vi "Reef Tele Align.vi"(1 "Robot Velocities":T2={"X Velocity"=-0.05891453742478221, "Y Velocity"=0.05531455287310416, "Rotational \nVelocity"=-0.0}, 2 "PigeonIMUDevRef":T3={"DeviceStatus"={"status"=FALSE, "code"=0, "source"=""}, "Device Number"=21, "Type"=352321536, "Device ID"=352321557, "Handle"=27000480, "UsageFrame"=0, "Library Path"=path "libCTRE_PhoenixCCI.so"} {"Type" items=["CAN"=352321536, "TalonSRX"=33554432]}) -> (0 "Robot Velocities":T2={"X Velocity"=-0.05891453742478221, "Y Velocity"=0.05531455287310416, "Rotational \nVelocity"=-0.0})   [LabVIEW 2023]
uses:
  <vilib>/Rock Robotics/WPI/ThirdParty/Phoenix-LabVIEW/Pigeon IMU/CTRE_PigeonIMU_DeviceRef.ctl
  <vilib>/Rock Robotics/WPI/ThirdParty/Phoenix-LabVIEW/Pigeon IMU/CTRE_PigeonIMU_ConnectionType.ctl
  swerve/Type Definitions/Data/Robot Velocities.ctl
  <vilib>/Rock Robotics/Network Tables/NT Read Numeric Array.vi
  <vilib>/Rock Robotics/WPI/ThirdParty/Phoenix-LabVIEW/Pigeon IMU/CTRE_PigeonIMU_GetYPR.vi
panel:
  in  "F Value X":dbl=0.8 format="%.2f"
  in  "FeedFwd Value":dbl=0.8 format="%.2f"
  out "Limelight Value":dbl[](array[numeric])=[0.09069335352360994, 0.2555777244634621, -1.0504762124767997, -1.0032725806064795, -8.759387018378728, -0.17873698055030388]
  in  "Setpoint Y":dbl=1.0
  in  "Setpoint X":dbl
  in  "Deadband Y":dbl=0.1
  in  "PID Y":T1={"proportional gain (Kp)"=0.2, "integral time (Ki)"=0.0, "derivative time (Kd)"=0.0} {"derivative time (Kd)" format="%.3f"; "integral time (Ki)" format="%.3f"; "proportional gain (Kp)" format="%.3f"}
  out "Err/Out Chart 2":cluster{dbl, dbl}(graph)={2.1086785037111793, 0.6326035511133538}
  out "SP/PV Chart 2":cluster{"setpoint":dbl, "process variable":dbl}(graph)={"setpoint"=1.0, "process variable"=-1.1086785037111793}
  out "SP/PV Chart":cluster{"setpoint":dbl, "process variable":dbl}(graph)={"setpoint"=0.0, "process variable"=0.10840384468168587}
  out "Err/Out Chart":cluster{dbl, dbl}(graph)={-0.10840384468168587, -0.03252115340450576}
  in  "PID X":T1={"proportional gain (Kp)"=0.2, "integral time (Ki)"=0.0, "derivative time (Kd)"=0.0} {"derivative time (Kd)" format="%.3f"; "integral time (Ki)" format="%.3f"; "proportional gain (Kp)" format="%.3f"}
  in  "Deadband X":dbl=0.075
  out "Yaw Pitch Roll":cluster{"Yaw":dbl, "Pitch":dbl, "Roll":dbl}
  out "X":dbl=0.09069335352360994
  out "Y":dbl=-1.0504762124767997
  # "Y Errors"
  # "X Errors"
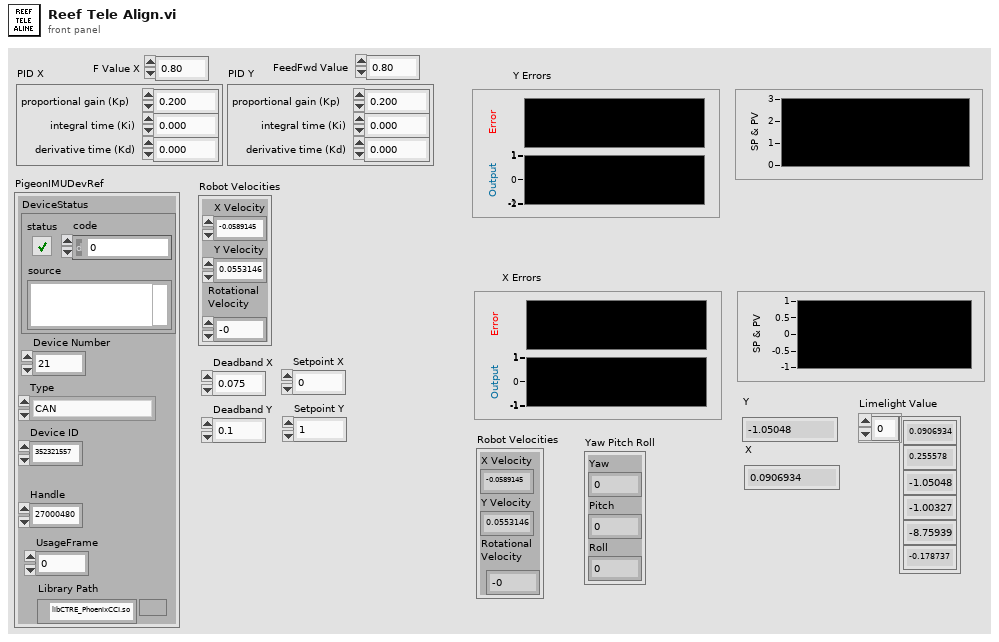
[diagram p1: front panel]
types:
  T1 = cluster{"proportional gain (Kp)":dbl, "integral time (Ki)":dbl, "derivative time (Kd)":dbl}
  T2 = typedef "Robot Velocities.ctl" = cluster{"X Velocity":dbl, "Y Velocity":dbl, "Rotational \nVelocity":dbl}
  T3 = typedef "CTRE_PigeonIMU_DeviceRef.ctl" = cluster{"DeviceStatus":errorcluster, "Device Number":u8, "Type":T4, "Device ID":u32, "Handle":u64, "UsageFrame":u32, "Library Path":path}
  T4 = typedef "CTRE_PigeonIMU_ConnectionType.ctl" = u32
  T5 = cluster{"value[0]":dbl, "value[1]":dbl, "value[2]":dbl, "value[3]":dbl, "value[4]":dbl, "value[5]":dbl, "value[6]":dbl, "value[7]":dbl, "value[8]":dbl}
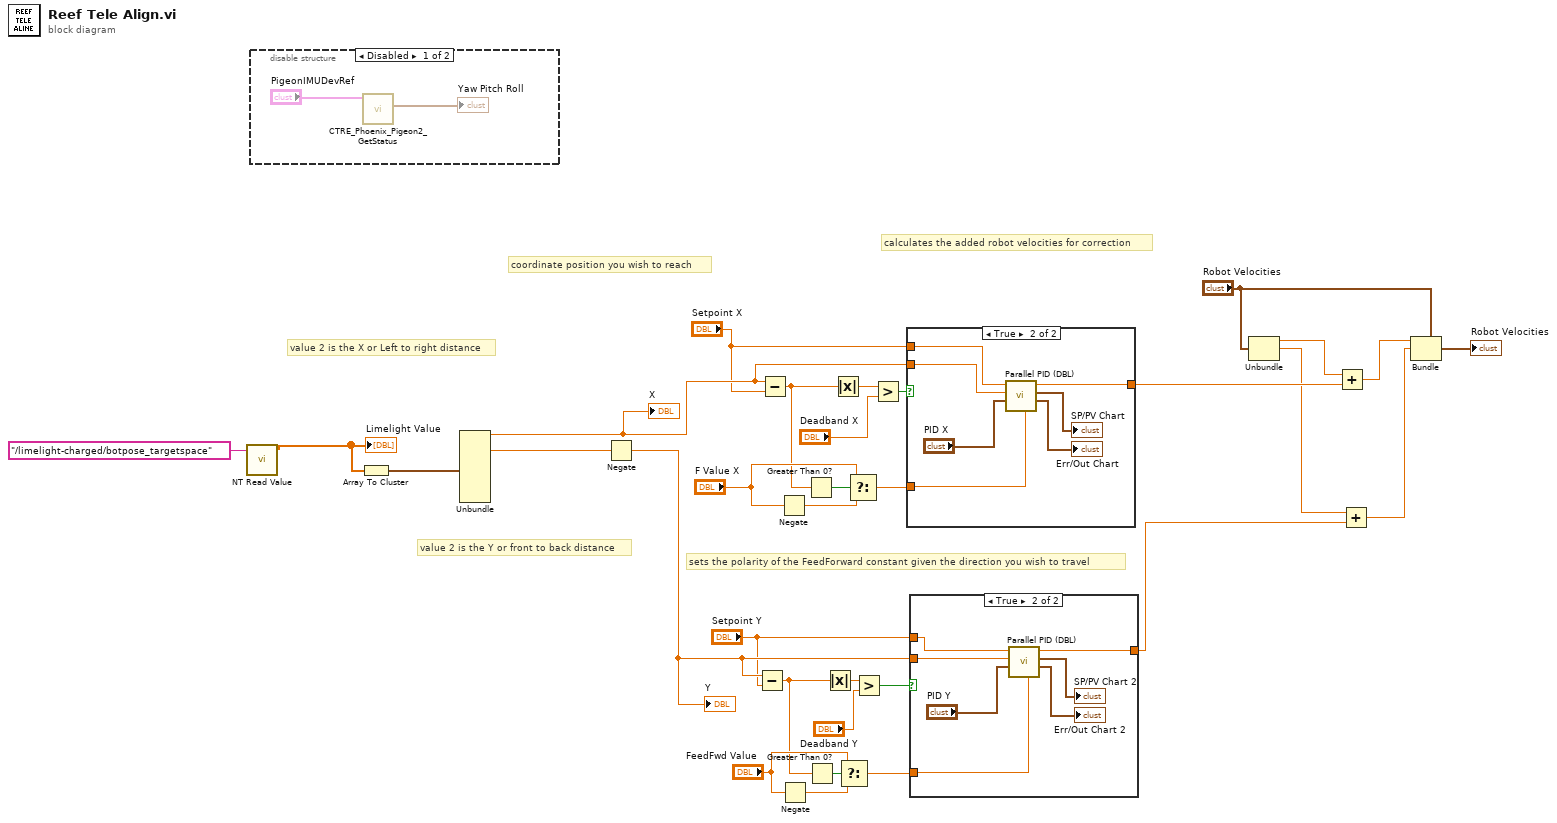
[diagram p0: block diagram]
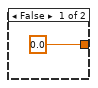
[diagram p2: hidden frame]
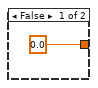
[diagram p3: hidden frame]
diagram:
  # "calculates the added robot velocities for correction"
  # "sets the polarity of the FeedForward constant given the direction you wish to travel"
  # "coordinate position you wish to reach"
  # "value 2 is the X or Left to right distance"
  # "value 2 is the Y or front to back distance"
  n1 = call-poly <vilib>:"NT Read Value.vi"("name"="/limelight-charged/botpose_targetspace") -> ("value"=w23:dbl[])  [unwired: 8 in, 2 out]
  "Limelight Value" <- w23
  n2 = disable-structure shown="Disabled" {
    frame Disabled {
      n3 = call-poly <vilib>:"CTRE_Phoenix_Pigeon2_GetStatus.vi"("PigeonIMUDevRef"="PigeonIMUDevRef") -> ("Yaw Pitch Roll"=→"Yaw Pitch Roll":cluster{"Yaw":dbl, "Pitch":dbl, "Roll":dbl})  [unwired: 8 in, 2 out]
    }
    frame Enabled {
    }
  }
  n4 = Array To Cluster(array=w23) -> (cluster=w22:T5)
  n5 = Unbundle(w22) -> ("value[0]"=w11:dbl, "value[2]"=w21:dbl)  [unwired: 7 out]
  "X" <- w11
  n6 = Negate(x=w21) -> (-x=w20:dbl)
  "Y" <- w20
  n7 = Subtract(x=w20, y="Setpoint Y") -> (x-y=w2:dbl)
  n8 = Subtract(x=w11, y="Setpoint X") -> (x-y=w12:dbl)
  n9 = Negate(x="F Value X") -> (-x=w16:dbl)
  n10 = Negate(x="FeedFwd Value") -> (-x=w3:dbl)
  n11 = Greater Than 0?(x=w12) -> (x > 0?=w18:bool)
  n12 = Greater Than 0?(x=w2) -> (x > 0?=w5:bool)
  n13 = Absolute Value(x=w2) -> (abs(x)=w6:dbl)
  n14 = Absolute Value(x=w12) -> (abs(x)=w19:dbl)
  n15 = Select(t="FeedFwd Value", s=w5, f=w3) -> (s? t:f=w1:dbl)
  n16 = Select(t="F Value X", s=w18, f=w16) -> (s? t:f=w13:dbl)
  n17 = Greater?(x=w6, y="Deadband Y") -> (0:w9:bool)
  n18 = Greater?(x=w19, y="Deadband X") -> (0:w14:bool)
  n19 = case shown="True" w14 {
    tunnel: [0.0 ("output") w41] -> w28
    tunnel: w13 -> [_ w38]
    tunnel: w11 -> [_ w36]
    tunnel: "Setpoint X" -> [_ w37]
    frame False {
    }
    frame True {
      n20 = call <vilib>:"Parallel PID (DBL).vi"("FeedFwd Value"=w38, "PID gains"="PID X", "process variable"=w36, "setpoint"=w37) -> ("Err/Out Chart"=→"Err/Out Chart":cluster{dbl, dbl}, "SP/PV Chart"=→"SP/PV Chart":cluster{"setpoint":dbl, "process variable":dbl}, "output"=w41:dbl)  [unwired: 4 in, 1 out]
    }
  }
  n21 = case shown="True" w9 {
    tunnel: w20 -> [_ w50]
    tunnel: [0.0 ("output") w48] -> w25
    tunnel: "Setpoint Y" -> [_ w45]
    tunnel: w1 -> [_ w44]
    frame False {
    }
    frame True {
      n22 = call <vilib>:"Parallel PID (DBL).vi"("FeedFwd Value"=w44, "PID gains"="PID Y", "process variable"=w50, "setpoint"=w45) -> ("Err/Out Chart"=→"Err/Out Chart 2":cluster{dbl, dbl}, "SP/PV Chart"=→"SP/PV Chart 2":cluster{"setpoint":dbl, "process variable":dbl}, "output"=w48:dbl)  [unwired: 4 in, 1 out]
    }
  }
  n23 = Unbundle("Robot Velocities") -> ("X Velocity"=w29:dbl, "Y Velocity"=w27:dbl)  [unwired: 1 out]
  n24 = Add(x=w29, y=w28) -> (x+y=w30:dbl)
  n25 = Add(x=w27, y=w25) -> (x+y=w26:dbl)
  n26 = Bundle(cluster="Robot Velocities", "X Velocity"=w30, "Y Velocity"=w26) -> (→"Robot Velocities":T2)  [unwired: 1 in]
